vi "Eq.vi"(1 "Equivalent Nozzle Radius (Rn)":dbl, 2 "Nozzle Area (An)":dbl, 3 "Vehicle Frontal Area (Am)":dbl, 4 "Nozzle-source point (Xs)":dbl) -> (0 "Nozzle Blockage Factor (Eq)":dbl)   [LabVIEW 2017]
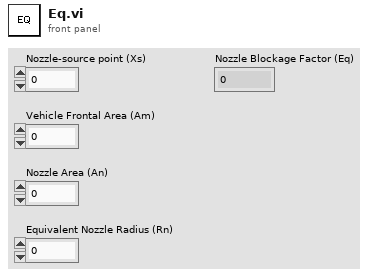
[diagram p1: front panel]
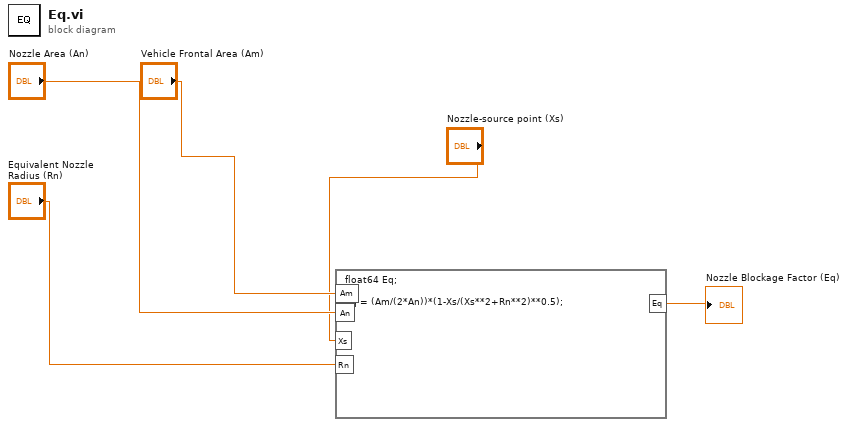
[diagram p0: block diagram]
diagram:
  n1 = formula code="float64 Eq; \n\nEq = (Am/(2*An))*(1-Xs/(Xs**2+Rn**2)**0.5);"("Am"="Vehicle Frontal Area (Am)", "An"="Nozzle Area (An)", "Xs"="Nozzle-source point (Xs)", "Rn"="Equivalent Nozzle Radius (Rn)") -> ("Eq"=→"Nozzle Blockage Factor (Eq)":dbl)
